vi "Draw Characters.vi"(8 "error in (no error)":errorcluster, 9 "Move Data":cluster{"Direction":T2, "Step (px)":u16}[](array[cluster]), 10 "Picture In":T1, 11 "Draw in":refnum<class "Draw.lvclass">) -> (0 "error out":errorcluster, 2 "Picture Out":T1, 3 "Draw out":refnum<class "Draw.lvclass">)   [LabVIEW 2016, in "PacManClasses.lvlib" / "Draw.lvclass"]
uses:
  Draw.lvclass
  Generic Controls/Picture.ctl
  Generic Controls/Direction.ctl
  Geometric Figure/UI Object.lvclass
  PacManClasses.lvlib
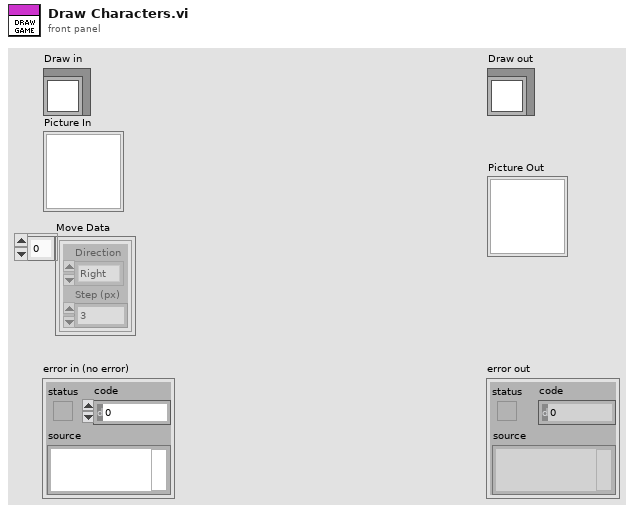
[diagram p1: front panel]
types:
  T1 = typedef "PacManClasses.lvlib/Picture.ctl" = picture
  T2 = typedef "PacManClasses.lvlib/Direction.ctl" = enum16{"Up", "Down", "Left", "Right"}
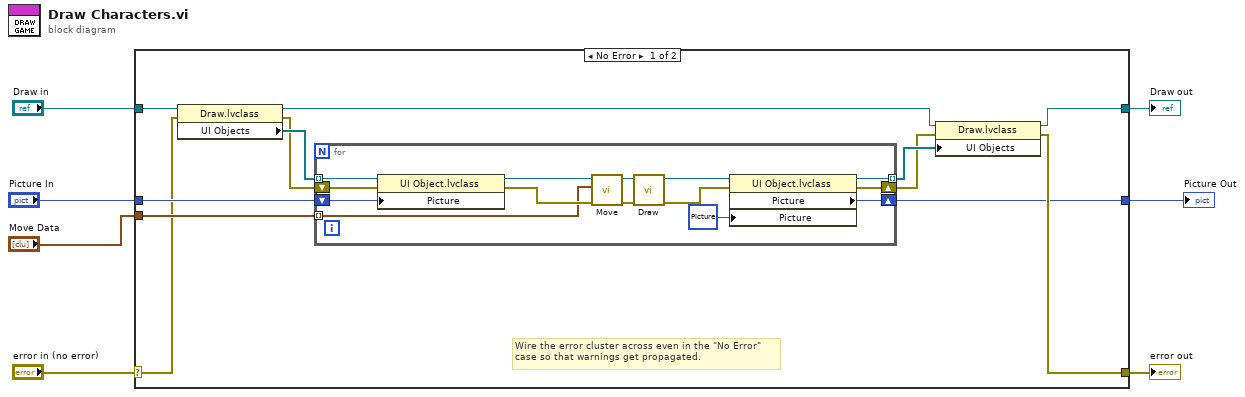
[diagram p0: block diagram]
diagram:
  n1 = case shown="No Error" "error in (no error)" {
    selector: "error in (no error)" -> [w14 w36]
    tunnel: [w10 w36] -> w6
    tunnel: [w9 w35] -> w4
    tunnel: "Draw in" -> [w19 w35]
    tunnel: "Picture In" -> [w17 w34]
    tunnel: "Move Data" -> [w15 _]
    tunnel: [w8 w34] -> w1
    frame No Error {
      # "Wire the error cluster across even in the \"No Error\"\ncase so that warnings get propagated."
      n2 = property class="Draw.lvclass"(reference=w19, error in=w14) -> (reference out=w12:refnum<class "Draw.lvclass">, error out=w16:errorcluster, "UI Objects"=w18:refnum<class "UI Object.lvclass">[])
      n3 = for {
        tunnel: w18 -> [w29] mode=indexing
        shift-right: [w22] -> w8
        shift-left: w17 -> [w27]
        shift-right: [w23] -> w11
        shift-left: w16 -> [w26]
        tunnel: w15 -> [w24] mode=indexing
        tunnel: [w21] -> w13 mode=indexing
        n4 = property class="UI Object.lvclass"(reference=w29, error in=w26, "Picture"=w27) -> (reference out=w28:refnum<class "UI Object.lvclass">, error out=w25:errorcluster)
        n5 = call-dynamic "Move.vi"("error in (no error)"=w25, "Move Data"=w24, "Geometric Figure in"=w28) -> ("error out"=w32:errorcluster, "Geometric Figure out"=w33:refnum<class "UI Object.lvclass">)  [unwired: 7 in]
        n6 = call-dynamic "Draw.vi"("error in (no error)"=w32, "Geometric Figure in"=w33) -> ("error out"=w31:errorcluster, "Geometric Figure out"=w30:refnum<class "UI Object.lvclass">)  [unwired: 8 in]
        n7 = property class="UI Object.lvclass"(reference=w30, error in=w31, "Picture"=T1 data[5B]) -> (reference out=w21:refnum<class "UI Object.lvclass">, error out=w23:errorcluster, "Picture"=w22:T1)
      }
      n8 = property class="Draw.lvclass"(reference=w12, error in=w11, "UI Objects"=w13) -> (reference out=w9:refnum<class "Draw.lvclass">, error out=w10:errorcluster)
    }
    frame Error {
    }
  }
  "error out" <- w6
  "Draw out" <- w4
  "Picture Out" <- w1
